vi "OpenGrayImg.vi"(1 "Image Name":string, 2 "Img Path":path) -> (0 "Image Out":T1)   [LabVIEW 2014]
uses:
  <vilib>/vision/Image Controls.llb/IMAQ Image.ctl
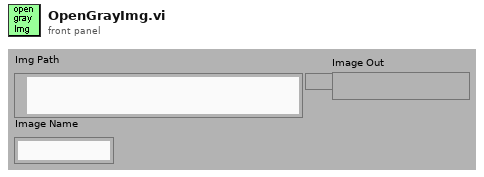
[diagram p1: front panel]
types:
  T1 = typedef "IMAQ Image.ctl" = refnum<image>
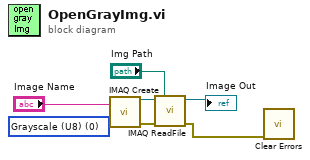
[diagram p0: block diagram]
diagram:
  w2 = u32 0 items=["Grayscale (U8)", "Grayscale (I16)", "Grayscale (SGL)", "Complex (CSG)", "RGB (U32)", "HSL (U32)", "RGB (U64)"] ("Image Type")
  n1 = call "IMAQ Create"("Image Name"="Image Name", "Image Type"=w2) -> ("New Image"=w4:T1, "error out"=w3:errorcluster)  [unwired: 2 in, 1 out]
  n2 = call "IMAQ ReadFile"("File Path"="Img Path", "error in (no error)"=w3, "Image"=w4) -> ("error out"=w1:errorcluster, "Image Out"=→"Image Out":T1)  [unwired: 2 in, 5 out]
  n3 = call <vilib>:"Clear Errors.vi"("error in (no error)"=w1) -> ()  [unwired: 5 in, 2 out]
